vi "FindProperties.vi"(8 "error in (no error)":errorcluster, 11 "CS in":refnum<class "CS.lvclass">) -> (0 "error out":errorcluster, 3 "CS out":refnum<class "CS.lvclass">)   [LabVIEW 2013, in "CS.lvclass"]
uses:
  CS.lvclass
  baseClass/baseClass.lvclass
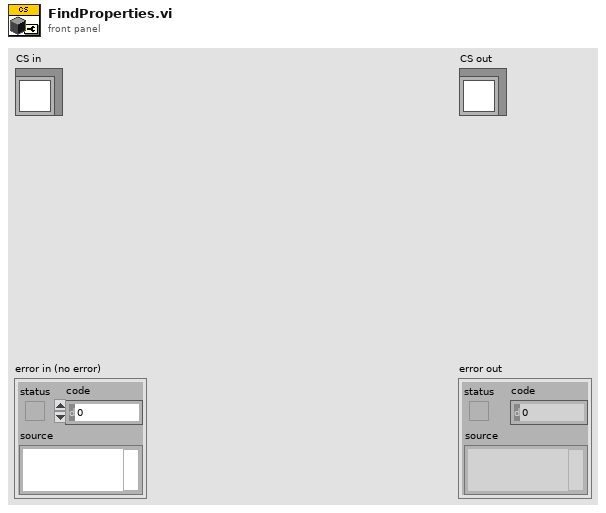
[diagram p1: front panel]
types:
  T1 = typedef "baseClass.lvclass/propertyDef.ctl" = cluster{"Name":string, "types":T2, "UserDefined":string, "Array":bool}
  T2 = typedef "baseClass.lvclass/types.ctl" = enum16{"String", "Int32", "Uint32", "Array", "Class", "Double", "Enum"}
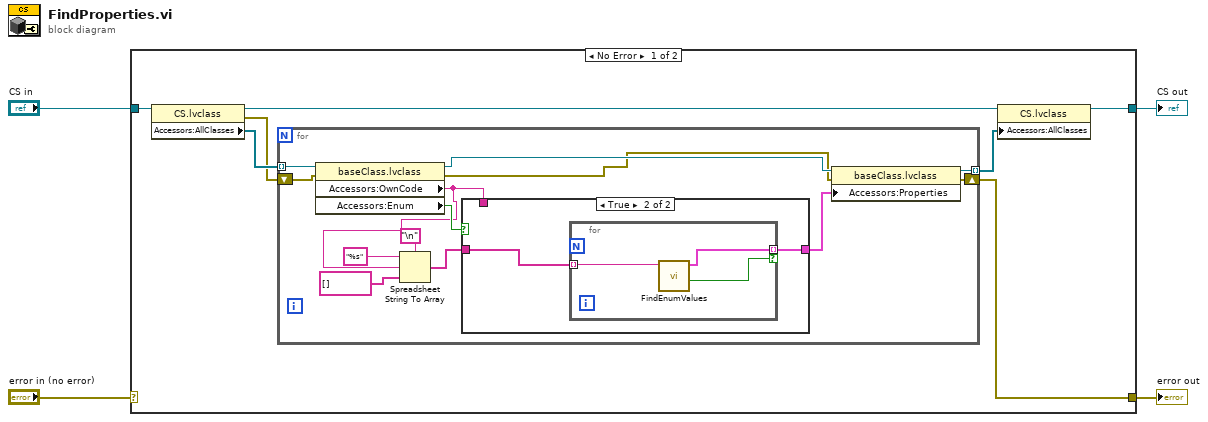
[diagram p0: block diagram]
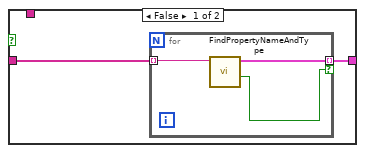
[diagram p2: hidden frame]
diagram:
  n1 = case shown="No Error" "error in (no error)" {
    selector: "error in (no error)" -> [_ w36]
    tunnel: [w7 w36] -> w3
    tunnel: [w6 w35] -> w1
    tunnel: "CS in" -> [w11 w35]
    frame No Error {
      n2 = property class="CS.lvclass"(reference=w11) -> (reference out=w10:refnum<class "CS.lvclass">, error out=w8:errorcluster, "Accessors:AllClasses"=w9:refnum<class "baseClass.lvclass">[])  [unwired: 1 in]
      n3 = for {
        tunnel: w9 -> [w24] mode=indexing
        tunnel: [w21] -> w5 mode=indexing
        shift-right: [w20] -> w7
        shift-left: w8 -> [w19]
        n4 = property class="baseClass.lvclass"(reference=w24, error in=w19) -> (reference out=w23:refnum<class "baseClass.lvclass">, error out=w18:errorcluster, "Accessors:OwnCode"=w13:string, "Accessors:Enum"=w17:bool)
        n5 = Spreadsheet String To Array(delimiter (Tab)="\n", format string="%s", spreadsheet string=w13, array type (2D Dbl)=string[] []) -> (array=w12:string[])
        n6 = case shown="True" w17 {
          tunnel: w13 -> [_ _]
          tunnel: [w26 w30] -> w22
          tunnel: w12 -> [w25 w31]
          frame False {
            n7 = for {
              tunnel: w25 -> [w29] mode=indexing
              tunnel: [w27] -> w26 mode=indexing if=w28
              n8 = call "FindPropertyNameAndType.vi"("string"=w29) -> ("PropertyFound"=w28:bool, "properties"=w27:T1)  [unwired: 9 in]
            }
          }
          frame True {
            n9 = for {
              tunnel: w31 -> [w34] mode=indexing
              tunnel: [w33] -> w30 mode=indexing if=w32
              n10 = call "FindEnumValues.vi"("string"=w34) -> ("PropertyFound"=w32:bool, "properties"=w33:T1)  [unwired: 9 in]
            }
          }
        }
        n11 = property class="baseClass.lvclass"(reference=w23, error in=w18, "Accessors:Properties"=w22) -> (reference out=w21:refnum<class "baseClass.lvclass">, error out=w20:errorcluster)
      }
      n12 = property class="CS.lvclass"(reference=w10, "Accessors:AllClasses"=w5) -> (reference out=w6:refnum<class "CS.lvclass">)  [unwired: 1 in, 1 out]
    }
    frame Error {
    }
  }
  "error out" <- w3
  "CS out" <- w1
